vi "Read Module Init on Error.vi"(7 "Module ID":string, 8 "error in":errorcluster, 11 "Standard Engine Repo Data in":refnum<class "Standard Engine Configuration.lvclass">) -> (0 "error out":errorcluster, 2 "Initialize on Error?":bool, 3 "Standard Engine Repo Data out":refnum<class "Standard Engine Configuration.lvclass">)   [LabVIEW 2013, in "Standard Engine Configuration.lvclass"]
doc: "Returns the decimation values for the specified module that were configured using the 'Write Module Decimation.vi'."
uses:
  Standard Engine Configuration.lvclass
  Standard Engine Configuration.lvclass/Standard Engine Configuration.ctl
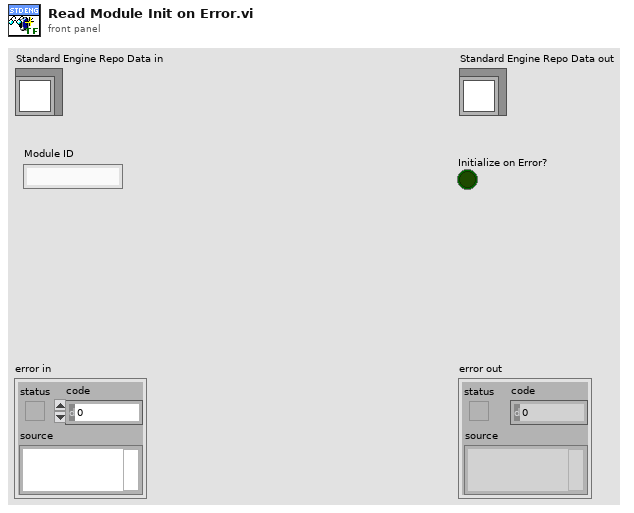
[diagram p1: front panel]
types:
  T1 = typedef "Standard Engine Configuration.lvclass/Module Specific Configuration.ctl" = cluster{"Module ID":string, "Module Decimation":T2, "error tag":string, "error responses":T3, "Initialize on Error?":bool}
  T2 = typedef "Standard Engine Configuration.lvclass/Module Decimation.ctl" = cluster{"Decimation":u16, "Offset":u16, "sort order":i32, "async?":bool}
  T3 = typedef "Standard Engine Configuration.lvclass/error responses.ctl" = cluster{"unknown":T4, "trivial":T4, "critical":T4, "recoverable":T4}
  T4 = typedef "Standard Engine Configuration.lvclass/error options.ctl" = cluster{"clear":bool, "notify":bool, "log":bool, "remove module":bool, "abort engine":bool, "go to safe state":bool, "recover module":bool}
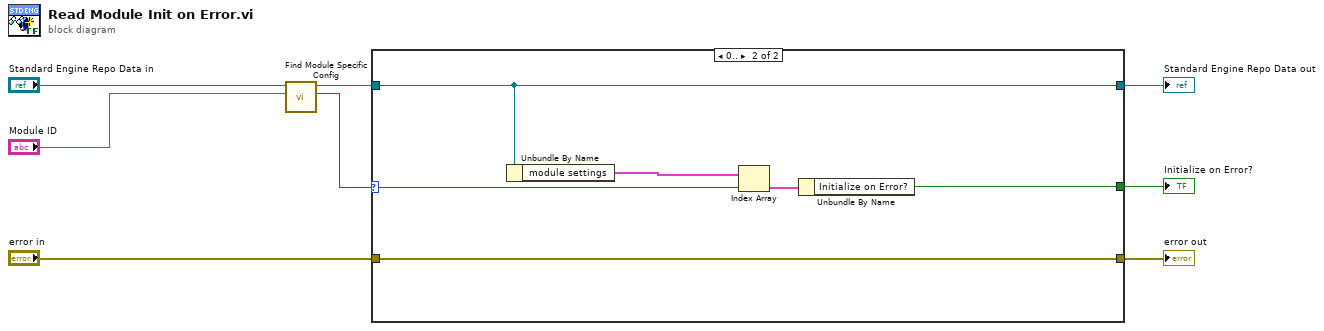
[diagram p0: block diagram]
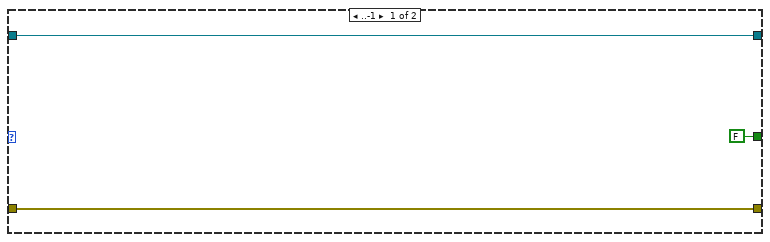
[diagram p2: hidden frame]
diagram:
  n1 = call "Find Module Specific Config.vi"("Module ID"="Module ID", "Standard Engine Repo Data in"="Standard Engine Repo Data in") -> ("Index"=w2:i32, "Standard Engine Repo Data out"=w3:refnum<class "Standard Engine Configuration.lvclass">)  [unwired: 8 in]
  n2 = case shown="0.." w2 {
    selector: w2 -> [_ w14]
    tunnel: w3 -> [w11 w15]
    tunnel: [FALSE ("Initialize on Error?") w12] -> w1
    tunnel: "error in" -> [w10 w13]
    tunnel: [w10 w13] -> w4
    tunnel: [w11 w15] -> w6
    frame ..-1 {
    }
    frame 0.. {
      n3 = Unbundle By Name(w15) -> ("module settings"=w17:T1[])
      n4 = Index Array(array=w17, index=w14) -> (element=w16:T1)
      n5 = Unbundle By Name(w16) -> ("Initialize on Error?"=w12:bool)
    }
  }
  "error out" <- w4
  "Standard Engine Repo Data out" <- w6
  "Initialize on Error?" <- w1
